vi "Get_Contained_Symbol.vi"(8 "error in (no error)":errorcluster, 11 "IB_Tree_Item_Source_Folder_Sync in":refnum<class "IB_Tree_Item_Source_Folder_Sync.lvclass">) -> (0 "error out":errorcluster, 3 "symbol index":i32)   [LabVIEW 2020, in "IB_Tree_Item_Source_Folder_Sync.lvclass"]
uses:
  <vilib>/AppBuilder/IB_Classes/Tree_Item_Source_Folder_Sync/IB_Tree_Item_Source_Folder_Sync.lvclass
  <vilib>/AppBuilder/IB_Classes/Tree_Item_Source_Folder_Sync/IB_Tree_Item_Source_Folder_Sync.lvclass/IB_Tree_Item_Source_Folder_Sync.ctl
  <resource>/Framework/Providers/Builds/Installer/controls/IB_Tree_DefaultSymbols.ctl
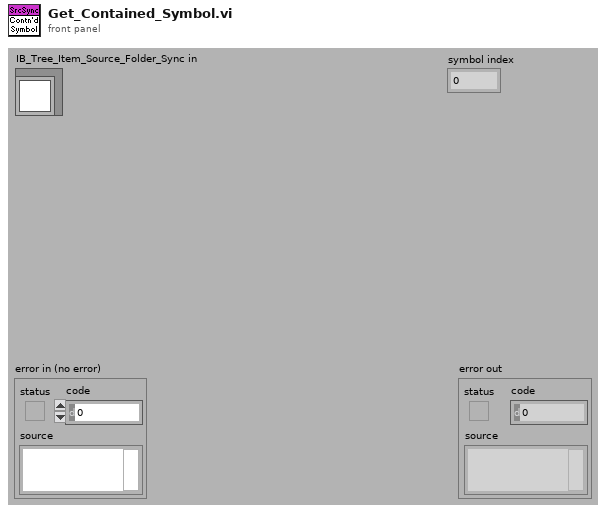
[diagram p1: front panel]
types:
  T1 = typedef "IB_Tree_DefaultSymbols.ctl" = enum16{"<unknown>", "closed folder", "open folder", "closed folder (default)", "open folder (default)", "closed sync folder", "open sync folder", "container folder", "my computer", "build specs", "exe", "dll", "source dist", "restful web service", ".net", "packed library", "c-generator", "target"}
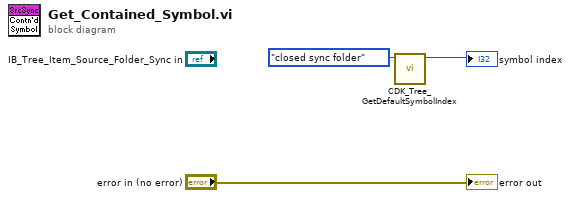
[diagram p0: block diagram]
diagram:
  n1 = call <resource>:"CDK_Tree_GetDefaultSymbolIndex.vi"("default symbol"=IB_Tree_DefaultSymbols."closed sync folder") -> ("symbol index"=→"symbol index":i32)  [unwired: 1 in, 9 out]
  "error out" <- "error in (no error)"
